vi "Create Destination.vi"(8 "Error In":errorcluster, 11 "For":T1(ring)=enum."Project (Visible)") -> (0 "Error Out":errorcluster, 3 "Destination":path=path "D:/Users/cfield/Code/Field R&D Services/Eulogy/Eulogy.lvproj/Eulogy/Hooks")   [LabVIEW 2018, in "Tools Menu.lvlib"]
uses:
  Tools Menu.lvlib
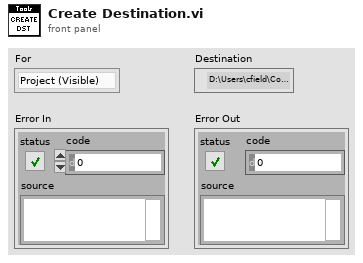
[diagram p1: front panel]
types:
  T1 = enum16{"System", "User", "Project (Visible)", "Project (Hidden)", "Custom..."}
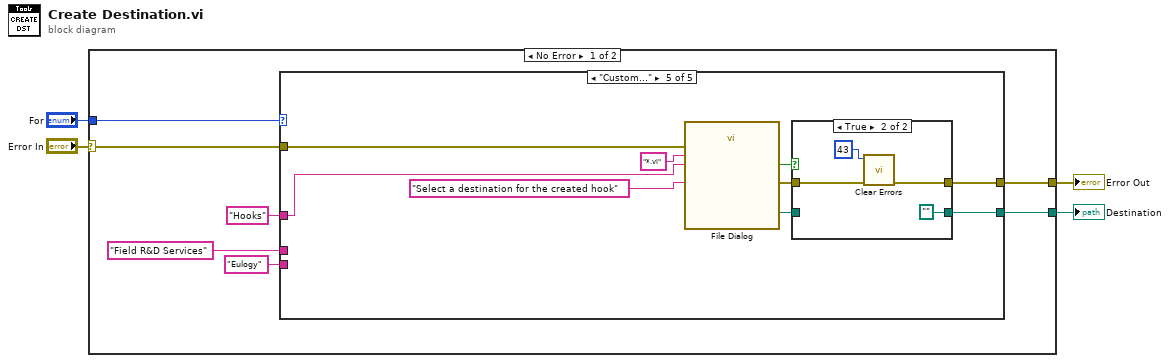
[diagram p0: block diagram]
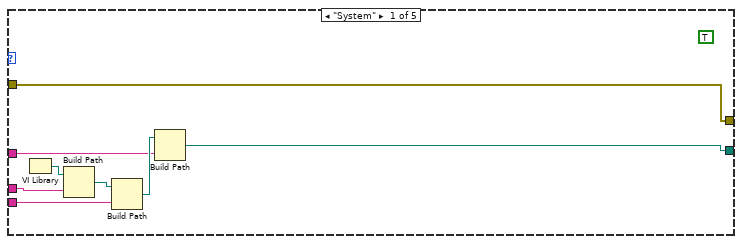
[diagram p2: hidden frame]
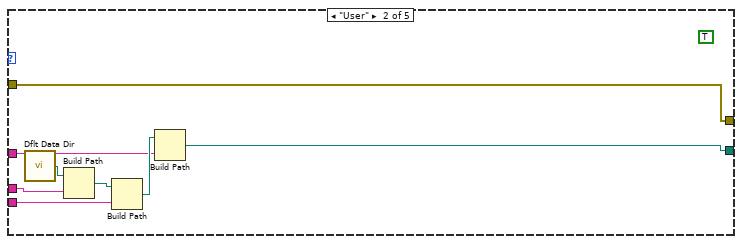
[diagram p3: hidden frame]
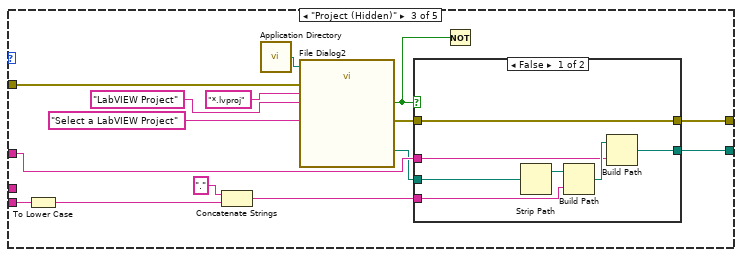
[diagram p4: hidden frame]
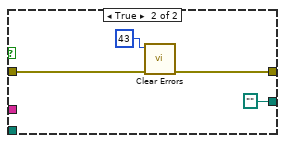
[diagram p5: hidden frame]
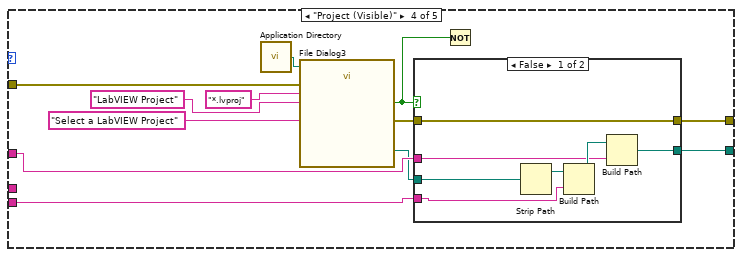
[diagram p6: hidden frame]
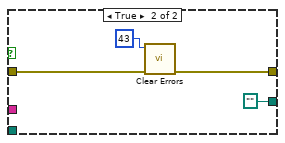
[diagram p7: hidden frame]
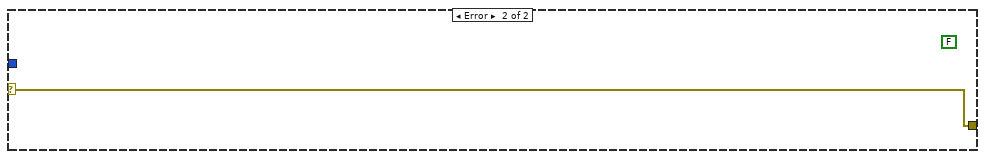
[diagram p9: hidden frame]
diagram:
  n1 = case shown="No Error" "Error In" {
    selector: "Error In" -> [w5 w92]
    tunnel: [w8 _] -> w4
    tunnel: [w7 w92] -> w3
    tunnel: "For" -> [w6 _]
    frame No Error {
      n2 = case shown="\"Custom...\"" w6 {
        tunnel: [w12 w20 w29 w56 w82] -> w7
        tunnel: [w16 w24 w42 w65 w80] -> w8
        tunnel: "Eulogy" ("name or relative path") -> [w15 w22 w40 w55 _]
        tunnel: "Field R&D Services" ("name or relative path") -> [w14 w23 _ _ _]
        tunnel: "Hooks" ("name or relative path") -> [w13 w21 w41 w64 w79]
        tunnel: w5 -> [w12 w20 w36 w63 w78]
        frame "System" {
          (unwired) TRUE
          n3 = VI Library() -> (path=w19:path)
          n4 = Build Path(base path=w19, name or relative path=w14) -> (appended path=w18:path)
          n5 = Build Path(base path=w18, name or relative path=w15) -> (appended path=w17:path)
          n6 = Build Path(base path=w17, name or relative path=w13) -> (appended path=w16:path)
        }
        frame "User" {
          (unwired) TRUE
          n7 = call <vilib>:"Dflt Data Dir.vi"() -> ("App:Default Data Directory"=w27:path)
          n8 = Build Path(base path=w27, name or relative path=w23) -> (appended path=w26:path)
          n9 = Build Path(base path=w26, name or relative path=w22) -> (appended path=w25:path)
          n10 = Build Path(base path=w25, name or relative path=w21) -> (appended path=w24:path)
        }
        frame "Project (Hidden)" {
          n11 = To Lower Case(string=w40) -> (all lower case string=w39:string)
          n12 = Concatenate Strings("." ("string"), w39) -> (w37:string)
          n13 = call <vilib>:"Application Directory.vi"() -> ("Application Directory"=w35:path)
          n14 = call "File Dialog2"("start path"=w35, "prompt"="Select a LabVIEW Project", "error in"=w36, "pattern (all files)"="*.lvproj", "pattern label"="LabVIEW Project") -> ("selected path"=w31:path, "cancelled"=w28:bool, "error out"=w30:errorcluster)  [unwired: 7 in, 1 out]
          n15 = case shown="False" w28 {
            tunnel: [w48 path ""] -> w42
            tunnel: w41 -> [w47 _]
            tunnel: w37 -> [w46 _]
            tunnel: w31 -> [w44 _]
            tunnel: w30 -> [w45 w53]
            tunnel: [w45 w51] -> w29
            frame False {
              n16 = Strip Path(path=w44) -> (stripped path=w43:path)  [unwired: 1 out]
              n17 = Build Path(base path=w43, name or relative path=w46) -> (appended path=w49:path)
              n18 = Build Path(base path=w49, name or relative path=w47) -> (appended path=w48:path)
            }
            frame True {
              n19 = call <vilib>:"Clear Errors.vi"("error in (no error)"=w53, "specific error code to clear (0: all)"=43) -> ("error out"=w51:errorcluster)  [unwired: 4 in, 1 out]
            }
          }
          n20 = Not(x=w28) -> ()  [unwired: 1 out]
        }
        frame "Project (Visible)" {
          n21 = call <vilib>:"Application Directory.vi"() -> ("Application Directory"=w62:path)
          n22 = call "File Dialog3"("start path"=w62, "prompt"="Select a LabVIEW Project", "error in"=w63, "pattern (all files)"="*.lvproj", "pattern label"="LabVIEW Project") -> ("selected path"=w58:path, "cancelled"=w54:bool, "error out"=w57:errorcluster)  [unwired: 7 in, 1 out]
          n23 = case shown="False" w54 {
            tunnel: [w71 path ""] -> w65
            tunnel: w64 -> [w70 _]
            tunnel: w55 -> [w69 _]
            tunnel: w58 -> [w67 _]
            tunnel: w57 -> [w68 w76]
            tunnel: [w68 w74] -> w56
            frame False {
              n24 = Strip Path(path=w67) -> (stripped path=w66:path)  [unwired: 1 out]
              n25 = Build Path(base path=w66, name or relative path=w69) -> (appended path=w72:path)
              n26 = Build Path(base path=w72, name or relative path=w70) -> (appended path=w71:path)
            }
            frame True {
              n27 = call <vilib>:"Clear Errors.vi"("error in (no error)"=w76, "specific error code to clear (0: all)"=43) -> ("error out"=w74:errorcluster)  [unwired: 4 in, 1 out]
            }
          }
          n28 = Not(x=w54) -> ()  [unwired: 1 out]
        }
        frame "Custom..." {
          n29 = call "File Dialog"("prompt"="Select a destination for the created hook", "error in"=w78, "pattern (all files)"="*.vi", "pattern label"=w79) -> ("selected path"=w81:path, "cancelled"=w77:bool, "error out"=w83:errorcluster)  [unwired: 8 in, 1 out]
          n30 = case shown="True" w77 {
            tunnel: w83 -> [w87 w91]
            tunnel: [w87 w89] -> w82
            tunnel: w81 -> [w86 _]
            tunnel: [w86 path ""] -> w80
            frame False {
            }
            frame True {
              n31 = call <vilib>:"Clear Errors.vi"("error in (no error)"=w91, "specific error code to clear (0: all)"=43) -> ("error out"=w89:errorcluster)  [unwired: 4 in, 1 out]
            }
          }
        }
      }
    }
    frame Error {
      (unwired) FALSE
    }
  }
  "Destination" <- w4
  "Error Out" <- w3
